vi "Check Close.vi"(8 "error in (no error)":errorcluster, 11 "Module in":refnum<class "Module.lvclass">) -> (0 "error out":errorcluster, 3 "Module out":refnum<class "Module.lvclass">)   [LabVIEW 2020, in "Volatus.lvlib" / "Module.lvclass"]
uses:
  Module.lvclass
  Module.lvclass/Module.ctl
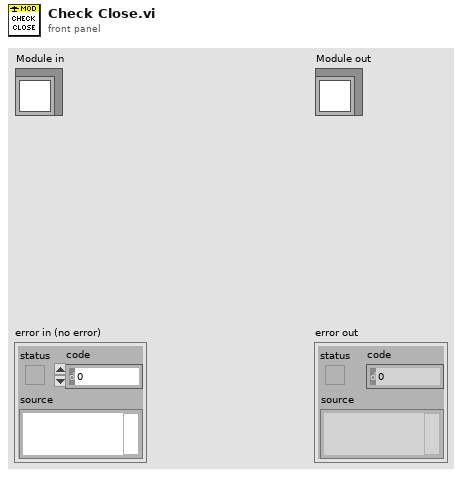
[diagram p1: front panel]
types:
  T1 = typedef "Volatus.lvlib/Module Status.ctl" = cluster{"MessageQ":refnum<class "MessageQ.lvclass">, "State":T2, "Hierarchy":string[]}
  T2 = typedef "Volatus.lvlib/Module.lvclass/State.ctl" = enum16{"Unknown", "Launched", "Starting", "Running", "Stopping", "Stopped", "Error - Starting", "Error - Run", "Error - Stopping"}
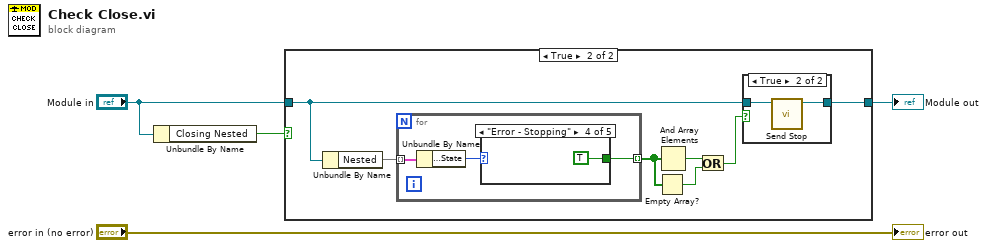
[diagram p0: block diagram]
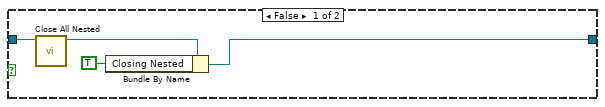
[diagram p2: hidden frame]
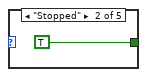
[diagram p5: hidden frame]
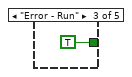
[diagram p6: hidden frame]
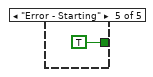
[diagram p7: hidden frame]
diagram:
  n1 = Unbundle By Name("Module in") -> ("Closing Nested"=w3:bool)
  n2 = case shown="True" w3 {
    tunnel: "Module in" -> [w8 w14]
    tunnel: [w6 w13] -> w2
    frame False {
      n3 = call "Close All Nested.vi"("Module in"=w8) -> ("Module out"=w7:refnum<class "Module.lvclass">)  [unwired: 9 in, 1 out]
      n4 = Bundle By Name(cluster=w7, "Closing Nested"=TRUE) -> (w6:refnum<class "Module.lvclass">)
    }
    frame True {
      n5 = Unbundle By Name(w14) -> ("Nested"=w15:map{refnum<class "MessageQ.lvclass">, T1})
      n6 = for {
        tunnel: w15 -> [w21] mode=indexing
        tunnel: [w19] -> w11 mode=indexing
        n7 = Unbundle By Name(w21) -> ("Status.State"=w20:T2)
        n8 = case shown="\"Error - Stopping\"" w20 {
          tunnel: [_ TRUE TRUE TRUE TRUE] -> w19
          frame Default {
          }
          frame "Stopped" {
          }
          frame "Error - Run" {
          }
          frame "Error - Stopping" {
          }
          frame "Error - Starting" {
          }
        }
      }
      n9 = Empty Array?(array=w11) -> (empty?=w9:bool)
      n10 = And Array Elements(Boolean array=w11) -> (logical AND=w12:bool)
      n11 = Or(x=w12, y=w9) -> (x .or. y?=w10:bool)
      n12 = case shown="True" w10 {
        tunnel: w14 -> [w16 w18]
        tunnel: [w16 w17] -> w13
        frame False {
        }
        frame True {
          n13 = call "Send Stop.vi"("Module in"=w18) -> ("Module out"=w17:refnum<class "Module.lvclass">)  [unwired: 9 in, 1 out]
        }
      }
    }
  }
  "Module out" <- w2
  "error out" <- "error in (no error)"
